vi "8-Axis (Manual).vi"() -> ()   [LabVIEW 2015]
uses:
  EMC API/EMC_Typedef_Motor_Parameters.ctl
  Typedef/Typedef_Motor_Action.ctl
  Functional_Global/Typedef_FPGA_Interface_Action.ctl
  <vilib>/Motion/Express/_s/nimc.ex.clearFaults.clearFaults.axis.vi
  <vilib>/Motion/Express/_s/nimc.ex.power.power.axis.vi
  <vilib>/Motion/Express/_s/nimc.ex.resetPosition.resetPosition.axis.vi
  <vilib>/Motion/Express/_s/nimc.ex.findReferenceMove.startReferenceMove.axis.modeReverseLimit.vi
  <vilib>/Motion/Express/_s/nimc.ex.findReferenceMove.startReferenceMove.axis.modeHome.vi
  <vilib>/Motion/Express/_s/nimc.ex.findReferenceMove.startReferenceMove.axis.modeForwardLimit.vi
  <vilib>/Motion/Express/_s/nimc.ex.read.readTrajectoryData.axis.vi
  <vilib>/Motion/Express/_s/nimc.ex.read.readMotionIO.axis.vi
  <vilib>/Motion/BlockNode/FB.NIMotion.xnode
panel:
  in  "velocity":dbl=1000.0
  in  "position[]":dbl[](array[numeric])=[5000.0, 5000.0, 5000.0, 5000.0, 5000.0, 5000.0, 5000.0, 5000.0]
  in  "resource":refnum<k21>="Axis 1"
  out "home active":bool
  out "rev. limit active":bool
  out "fwd. limit active":bool
  out "XY Graph":cluster{"X Array":dbl[], "Y Array":dbl[]}(graph)
  in  "interval":dbl=0.01 format="%#_13g"
  in  "Gear in/out":enum16{"Gear in", "Gear out"}(ring)
  in  "denominator":i32=1
  in  "numerator":i32=1
  in  "Master Axis":T1(ring)
  out "Array":dbl[](array[knob]) scale=0.0..1600.0
  in  "Clear Errors":bool
  in  "Command":T2
  in  "Motion Parameters":T3={"position"=1000.0, "velocity"=1000.0, "acceleration"=10000.0, "deceleration"=10000.0, "accel. jerk"=10000.0, "decel. jerk"=10000.0}
  in  "Axis Index":T1(ring)
  out "error":errorcluster
  out "Numeric":i32
  in  "Stop all motors":bool
  in  "Execute Command":bool
  in  "stop":bool
  out "Axis Velocities":T4(graph)
  out "Axis Positions":T4(graph)
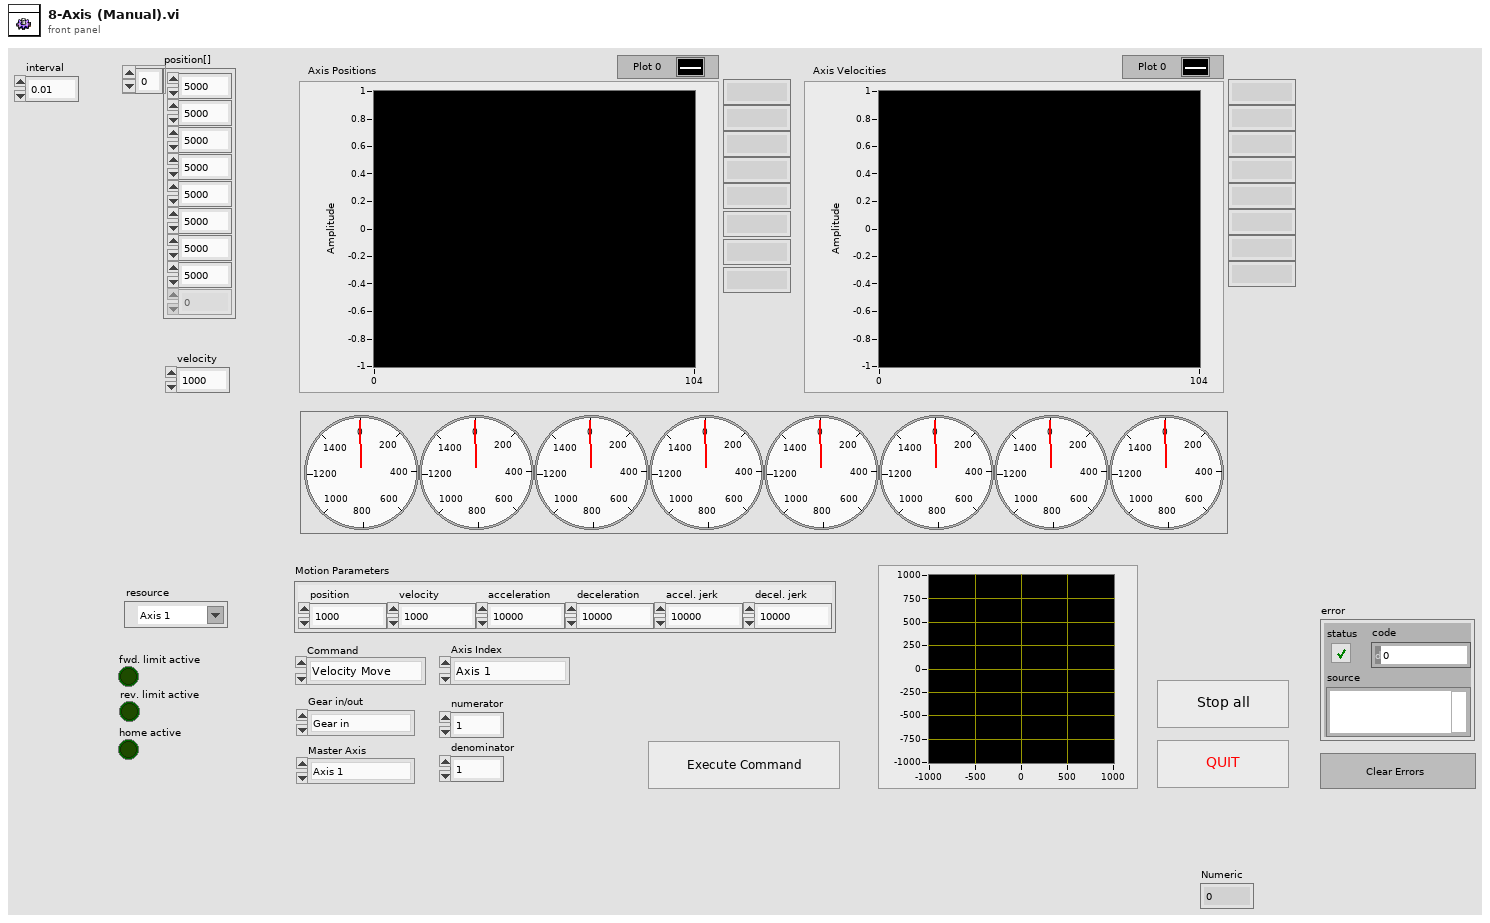
[diagram p1: front panel]
types:
  T1 = enum16{"Axis 1", "Axis 2", "Axis 3", "Axis 4", "Axis 5", "Axis 6", "Axis 7", "Axis 8"}
  T2 = typedef "Typedef_Motor_Action.ctl" = enum16{"Velocity Move", "REL Pos Move", "ABS Pos Move", "Stop", "Reset Position", "Coordinate_move", "Contour_move", "Gearing", "Find Fwd Limit", "Find Rev Limit", "Find Home"}
  T3 = typedef "EMC_Typedef_Motor_Parameters.ctl" = cluster{"position":dbl, "velocity":dbl, "acceleration":dbl, "deceleration":dbl, "accel. jerk":dbl, "decel. jerk":dbl}
  T4 = cluster{"[0]":dbl, "[1]":dbl, "[2]":dbl, "[3]":dbl, "[4]":dbl, "[5]":dbl, "[6]":dbl, "[7]":dbl}
  T5 = typedef "Typedef_FPGA_Interface_Action.ctl" = enum16{"Initialize FPGA", "Get FPGA Reference", "Close FPGA"}
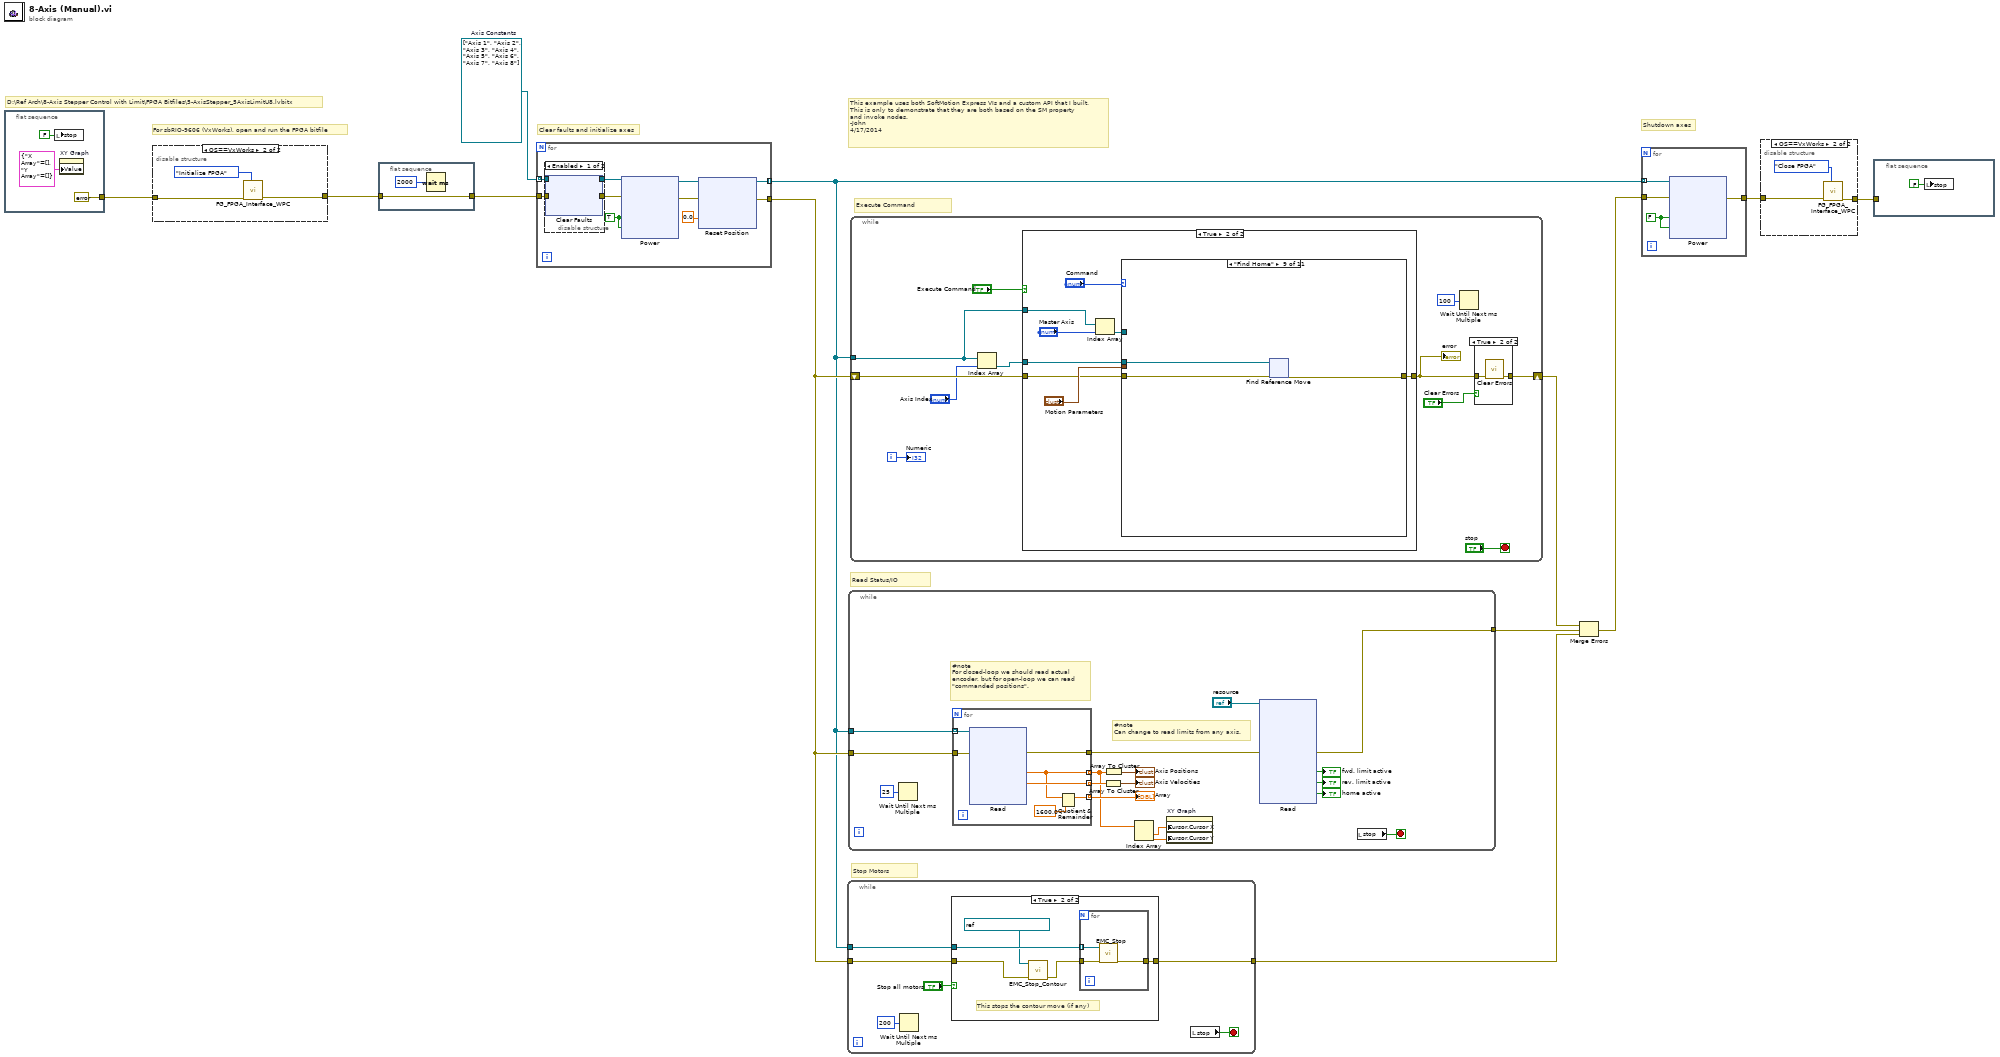
[diagram p0: block diagram]
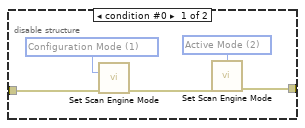
[diagram p3: hidden frame]
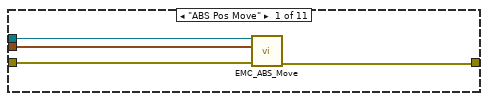
[diagram p8: hidden frame]
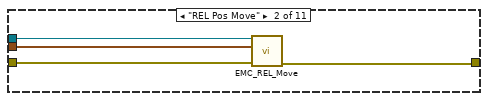
[diagram p9: hidden frame]
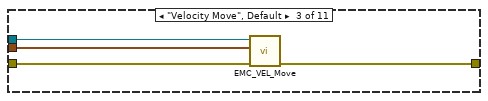
[diagram p10: hidden frame]
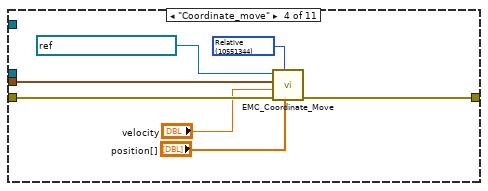
[diagram p11: hidden frame]
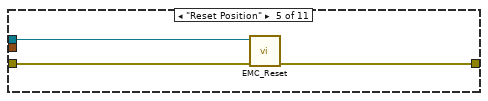
[diagram p12: hidden frame]
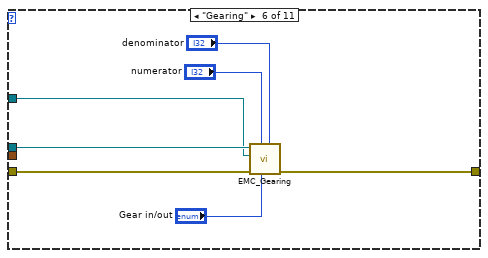
[diagram p13: hidden frame]
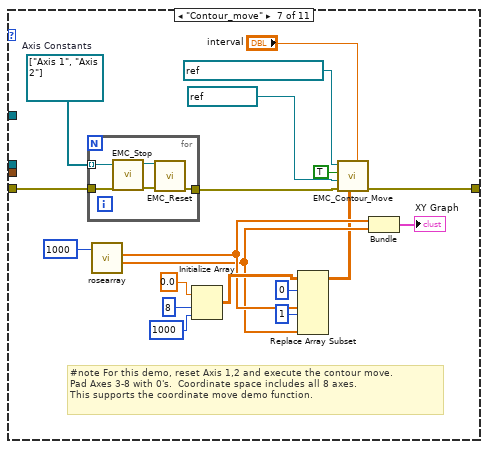
[diagram p14: hidden frame]
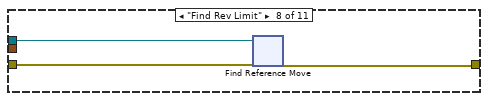
[diagram p15: hidden frame]
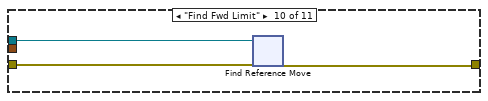
[diagram p16: hidden frame]
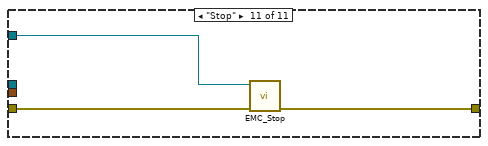
[diagram p17: hidden frame]
diagram:
  w11 = refnum<k21>[] ["Axis 1", "Axis 2", "Axis 3", "Axis 4", "Axis 5", "Axis 6", "Axis 7", "Axis 8"]  # Axis Constants
  # "For sbRIO-9606 (VxWorks), open and run the FPGA bitfile"
  # "D:\\Ref Arch\\8-Axis Stepper Control with Limit\\FPGA Bitfiles\\5-AxisStepper_5AxisLimitU8.lvbitx"
  # "Clear faults and initialize axes"
  # "This example uses both SoftMotion Express VIs and a custom API that I built.\nThis is only to demonstrate that they are both based on the SM property\nand invoke nodes. \n-John\n4/17/2014"
  # "Shutdown axes"
  # "Execute Command"
  # "Read Status/IO"
  # "Stop Motors"
  n1 = flat-sequence {
    tunnel: [errorcluster {"status"=FALSE, "code"=0, "source"=""} ("error in (no error)")] -> w8
    frame #0 {
      n2 = local write "stop"(FALSE ("stop")) -> ()
      n3 = property on="XY Graph" class="XYGraph (strict)"("Value"=cluster{"X Array":dbl[], "Y Array":dbl[]} {"X Array"=[], "Y Array"=[]} ("XY Graph")) -> ()  [unwired: 2 in, 2 out]
    }
  }
  n4 = disable-structure shown="OS==VxWorks" {
    disable-tunnel: [w20 w21] -> w2
    disable-tunnel: w8 -> [w19 w22]
    frame condition #0 {
      w16 = 1 items=["Configuration Mode"=1, "Active Mode"=2] ("mode (Active Mode)")
      w17 = 2 items=["Configuration Mode"=1, "Active Mode"=2] ("mode (Active Mode)")
      n5 = call <vilib>:"Set Scan Engine Mode.vi"("mode (Active Mode)"=w16, "error in (no error)"=w19) -> ("error out"=w18:errorcluster)  [unwired: 13 in]
      n6 = call <vilib>:"Set Scan Engine Mode.vi"("mode (Active Mode)"=w17, "error in (no error)"=w18) -> ("error out"=w20:errorcluster)  [unwired: 13 in]
    }
    frame condition #1 (active) {
      n7 = call "FG_FPGA_Interface_WPC.vi"("Action"=Typedef_FPGA_Interface_Action."Initialize FPGA", "error in"=w22) -> ("error out"=w21:errorcluster)  [unwired: 8 in, 1 out]
    }
  }
  n8 = flat-sequence {
    tunnel: w2 -> [w24]
    tunnel: [w24] -> w1
    frame #0 {
      n9 = Wait (ms)(milliseconds to wait=u32 2000) -> ()  [unwired: 1 out]
    }
  }
  n10 = for {
    tunnel: w11 -> [w29] mode=indexing
    tunnel: w1 -> [w28]
    tunnel: [w31] -> w5
    tunnel: [w30] -> w3 mode=indexing
    w35 = TRUE ("enable axis")
    n11 = disable-structure shown="Enabled" {
      disable-tunnel: w29 -> [w39 w45]
      disable-tunnel: w28 -> [w38 w44]
      disable-tunnel: [w37 w45] -> w27
      disable-tunnel: [w36 w44] -> w26
      frame Enabled {
        n12 = xnode ("Clear Faults")("resource"=w39, "error in"=w38) -> ("resource out"=w37:refnum<k21>, "error out"=w36:errorcluster)
      }
      frame Disabled {
      }
    }
    n13 = xnode ("Power")("enable axis"=w35, "enable drive"=w35, "resource"=w27, "error in"=w26) -> ("resource out"=w34:refnum<k21>, "error out"=w33:errorcluster)
    n14 = xnode ("Reset Position")("position"=0.0, "resource"=w34, "error in"=w33) -> ("resource out"=w30:refnum<k21>, "error out"=w31:errorcluster)
  }
  n15 = while {
    tunnel: w5 -> [w65]
    tunnel: w3 -> [w63]
    tunnel: [w61] -> w12
    stop <- w66 stop-if-true
    n16 = Wait Until Next ms Multiple(millisecond multiple=u32 200) -> ()  [unwired: 1 out]
    n17 = case shown="True" "Stop all motors" {
      tunnel: w65 -> [w67 w70]
      tunnel: [w67 w72] -> w61
      tunnel: w63 -> [_ w71]
      frame False {
      }
      frame True {
        # "This stops the contour move (if any)"
        n18 = call "EMC_Stop_Contour.vi"("error in (no error)"=w70, "coordinate"=refnum<k21> "Coordinate Space 1") -> ("error out"=w68:errorcluster)  [unwired: 9 in]
        n19 = for {
          tunnel: w68 -> [w75]
          tunnel: w71 -> [w73] mode=indexing
          tunnel: [w74] -> w72
          n20 = call "EMC_Stop.vi"("error in (no error)"=w75, "axis"=w73) -> ("error out"=w74:errorcluster)  [unwired: 8 in, 1 out]
        }
      }
    }
    n21 = local read "stop"() -> (w66:bool)
  }
  n22 = while {
    tunnel: w5 -> [w88]
    tunnel: w3 -> [w87]
    tunnel: [w76] -> w10
    stop <- w92 stop-if-true
    # "#note \nCan change to read limits from any axis."
    # "#note \nFor closed-loop we should read actual \nencoder, but for open-loop we can read\n\"commanded positions\"."
    n23 = Wait Until Next ms Multiple(millisecond multiple=u32 25) -> ()  [unwired: 1 out]
    n24 = for {
      tunnel: [w127] -> w78
      tunnel: [w122] -> w85 mode=indexing
      tunnel: [w126] -> w91 mode=indexing
      tunnel: w88 -> [w125]
      tunnel: w87 -> [w124] mode=indexing
      tunnel: [w121] -> w86 mode=indexing
      n25 = xnode ("Read")("resource"=w124, "error in"=w125) -> ("commanded position"=w122:dbl, "commanded vel."=w126:dbl, "error out"=w127:errorcluster)  [unwired: 2 out]
      n26 = Quotient & Remainder(x=w122, y=1600.0) -> (x-y*floor(x/y)=w121:dbl)  [unwired: 1 out]
    }
    "Array" <- w86
    n27 = Array To Cluster(array=w91) -> (cluster=→"Axis Velocities":T4)
    n28 = Array To Cluster(array=w85) -> (cluster=→"Axis Positions":T4)
    n29 = Index Array(array=w85) -> (element #1=w84:dbl, element #2=w83:dbl)  [unwired: 2 in]
    n30 = property on="XY Graph" class="XYGraph (strict)"("Cursor.Cursor X"=w84, "Cursor.Cursor Y"=w83) -> ()  [unwired: 2 in, 2 out]
    n31 = xnode ("Read")("resource"="resource", "error in"=w78) -> ("fwd. limit active"=→"fwd. limit active":bool, "rev. limit active"=→"rev. limit active":bool, "home active"=→"home active":bool, "error out"=w76:errorcluster)  [unwired: 6 out]
    n32 = local read "stop"() -> (w92:bool)
  }
  n33 = while {
    tunnel: w3 -> [w135]
    shift-right: [w136] -> w7
    shift-left: w5 -> [w140]
    i -> [w145]
    stop <- "stop" stop-if-true
    n34 = Index Array(array=w135, index="Axis Index") -> (element=w141:refnum<k21>)
    n35 = case shown="True" "Execute Command" {
      tunnel: w140 -> [w149 w156]
      tunnel: w141 -> [_ w155]
      tunnel: [w149 w154] -> w137
      tunnel: w135 -> [_ w151]
      frame False {
      }
      frame True {
        n36 = Index Array(array=w151, index="Master Axis") -> (element=w150:refnum<k21>)
        n37 = case shown="\"Find Home\"" "Command" {
          tunnel: "Motion Parameters" -> [w158 w162 w169 w170 _ _ _ _ _ _ _]
          tunnel: w156 -> [w161 w165 w168 w176 w179 w186 w198 w212 w231 w252 w272]
          tunnel: w155 -> [w159 w163 w167 _ w178 w185 _ w211 w230 w251 _]
          tunnel: [w160 w164 w166 w175 w177 w184 w205 w213 w232 w253 w271] -> w154
          tunnel: w150 -> [_ _ _ _ _ w180 _ _ _ _ w270]
          frame "ABS Pos Move" {
            n38 = call "EMC_ABS_Move.vi"("error in (no error)"=w161, "Motion Parameters"=w158, "axis"=w159) -> ("error out"=w160:errorcluster)  [unwired: 8 in]
          }
          frame "REL Pos Move" {
            n39 = call "EMC_REL_Move.vi"("error in (no error)"=w165, "Motion Parameters"=w162, "axis"=w163) -> ("error out"=w164:errorcluster)  [unwired: 8 in]
          }
          frame "Velocity Move", Default {
            n40 = call "EMC_VEL_Move.vi"("error in (no error)"=w168, "Motion Parameters"=w169, "axis"=w167) -> ("error out"=w166:errorcluster)  [unwired: 8 in]
          }
          frame "Coordinate_move" {
            w173 = 10551344 items=["Relative"=10551344, "Absolute"=10551337, "Relative To Capture"=10551345, "Velocity"=10551346, "Polyline"=11600101] ("line move mode")
            n41 = call "EMC_Coordinate_Move.vi"("position[]"="position[]", "line move mode"=w173, "error in (no error)"=w176, "velocity"="velocity", "Motion Parameters"=w170, "resource"=refnum<k21> "Coordinate Space 1") -> ("error out"=w175:errorcluster)  [unwired: 5 in]
          }
          frame "Reset Position" {
            n42 = call "EMC_Reset.vi"("error in (no error)"=w179, "axis"=w178) -> ("error out"=w177:errorcluster)  [unwired: 9 in]
          }
          frame "Gearing" {
            n43 = call "EMC_Gearing.vi"("denominator"="denominator", "Gear in/out"="Gear in/out", "numerator"="numerator", "error in (no error)"=w186, "master axis"=w180, "axis"=w185) -> ("error out"=w184:errorcluster)  [unwired: 5 in]
          }
          frame "Contour_move" {
            w196 = refnum<k21>[] ["Axis 1", "Axis 2"]  # Axis Constants
            # "#note For this demo, reset Axis 1,2 and execute the contour move.\nPad Axes 3-8 with 0's.  Coordinate space includes all 8 axes.\nThis supports the coordinate move demo function."
            n44 = for {
              tunnel: w198 -> [w209]
              tunnel: [w210] -> w197
              tunnel: w196 -> [w207] mode=indexing
              n45 = call "EMC_Stop.vi"("error in (no error)"=w209, "axis"=w207) -> ("error out"=w208:errorcluster, "axis out"=w206:refnum<k21>)  [unwired: 8 in]
              n46 = call "EMC_Reset.vi"("error in (no error)"=w208, "axis"=w206) -> ("error out"=w210:errorcluster)  [unwired: 9 in]
            }
            n47 = call "rosearray.vi"("Iterations"=u32 1000) -> ("Y Array"=w188:dbl[], "X Array"=w189:dbl[])  [unwired: 5 in, 1 out]
            n48 = Initialize Array(0.0 ("element"), 8 ("dimension size"), 1000 ("dimension size")) -> (w193:dbl[][])
            n49 = Replace Array Subset(array=w193, new element #1=w189, index (row) #1=0 ("index (row)"), new element #2=w188, index (row) #2=1 ("index (row)")) -> (w187:dbl[][])  [unwired: 2 in]
            n50 = call "EMC_Contour_Move.vi"("interval"="interval", "points[][]"=w187, "error in (no error)"=w197, "table"=refnum<k21> "Table 1" ("resource"), "overwrite"=TRUE, "coordinate"=refnum<k21> "Coordinate Space 1" ("resource")) -> ("error out"=w205:errorcluster)  [unwired: 5 in]
            n51 = Bundle("X Array"=w189, "Y Array"=w188) -> (→"XY Graph":cluster{"X Array":dbl[], "Y Array":dbl[]})  [unwired: 1 in]
          }
          frame "Find Rev Limit" {
            n52 = xnode "Find Reference Move"("resource"=w211, "error in"=w212) -> ("error out"=w213:errorcluster)  [unwired: 9 in, 2 out]
          }
          frame "Find Home" {
            n53 = xnode "Find Reference Move"("resource"=w230, "error in"=w231) -> ("error out"=w232:errorcluster)  [unwired: 11 in, 2 out]
          }
          frame "Find Fwd Limit" {
            n54 = xnode "Find Reference Move"("resource"=w251, "error in"=w252) -> ("error out"=w253:errorcluster)  [unwired: 9 in, 2 out]
          }
          frame "Stop" {
            n55 = call "EMC_Stop.vi"("error in (no error)"=w272, "axis"=w270) -> ("error out"=w271:errorcluster)  [unwired: 8 in, 1 out]
          }
        }
      }
    }
    "error" <- w137
    n56 = Wait Until Next ms Multiple(millisecond multiple=u32 100) -> ()  [unwired: 1 out]
    n57 = case shown="True" "Clear Errors" {
      tunnel: w137 -> [w146 w148]
      tunnel: [w146 w147] -> w136
      frame False {
      }
      frame True {
        n58 = call <vilib>:"Clear Errors.vi"("error in (no error)"=w148) -> ("error out"=w147:errorcluster)  [unwired: 5 in, 1 out]
      }
    }
    "Numeric" <- w145
  }
  n59 = Merge Errors(w7, w10, w12) -> (w4:errorcluster)
  n60 = for {
    tunnel: w3 -> [w276] mode=indexing
    tunnel: [w274] -> w6
    tunnel: w4 -> [w273]
    w275 = FALSE ("enable axis")
    n61 = xnode ("Power")("enable axis"=w275, "enable drive"=w275, "resource"=w276, "error in"=w273) -> ("error out"=w274:errorcluster)  [unwired: 1 out]
  }
  n62 = disable-structure shown="OS==VxWorks" {
    disable-tunnel: w6 -> [w287 w289]
    disable-tunnel: [w287 w288] -> w9
    frame condition #0 {
    }
    frame condition #1 (active) {
      n63 = call "FG_FPGA_Interface_WPC.vi"("Action"=Typedef_FPGA_Interface_Action."Close FPGA", "error in"=w289) -> ("error out"=w288:errorcluster)  [unwired: 8 in, 1 out]
    }
  }
  n64 = flat-sequence {
    tunnel: w9 -> [_]
    frame #0 {
      n65 = local write "stop"(FALSE ("stop")) -> ()
    }
  }
